vi "WinCI Open Project.vi"(8 "error in (no error)":errorcluster, 11 "configuration data":string) -> (0 "error out":errorcluster, 2 "status message":string, 3 "source control reference out":T1)   [LabVIEW 2017, in "NI_SCC_WinCI.lvlib"]
uses:
  <vilib>/SourceControl/Providers/WinCI/NI_SCC_WinCI.lvlib
  <vilib>/SourceControl/sccapi/SCCAPI Refnum.ctl
  <vilib>/SourceControl/support/SCCSup ConfigData Conv.ctl
  <vilib>/SourceControl/Providers/WinCI/WinCI SCC Project Details.ctl
  <vilib>/SourceControl/support/SCCSup Message Strings GLBL.vi
  <vilib>/SourceControl/sccapi/NI_SCC.lvlib
panel:
  out "returned project details":string
  in  "dummy refnum":T1
  out "result":i32
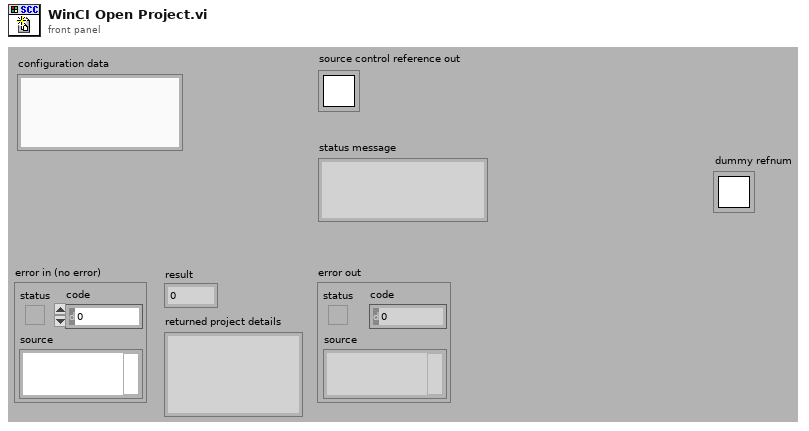
[diagram p1: front panel]
types:
  T1 = typedef "NI_SCC.lvlib/SCCAPI Refnum.ctl" = refnum<k1>
  T2 = typedef "SCCSup ConfigData Conv.ctl" = enum16{"from config data", "to config data"}
  T3 = typedef "NI_SCC_WinCI.lvlib/WinCI SCC Project Details.ctl" = cluster{"user name":string, "project name":string, "local path":string, "database name":string}
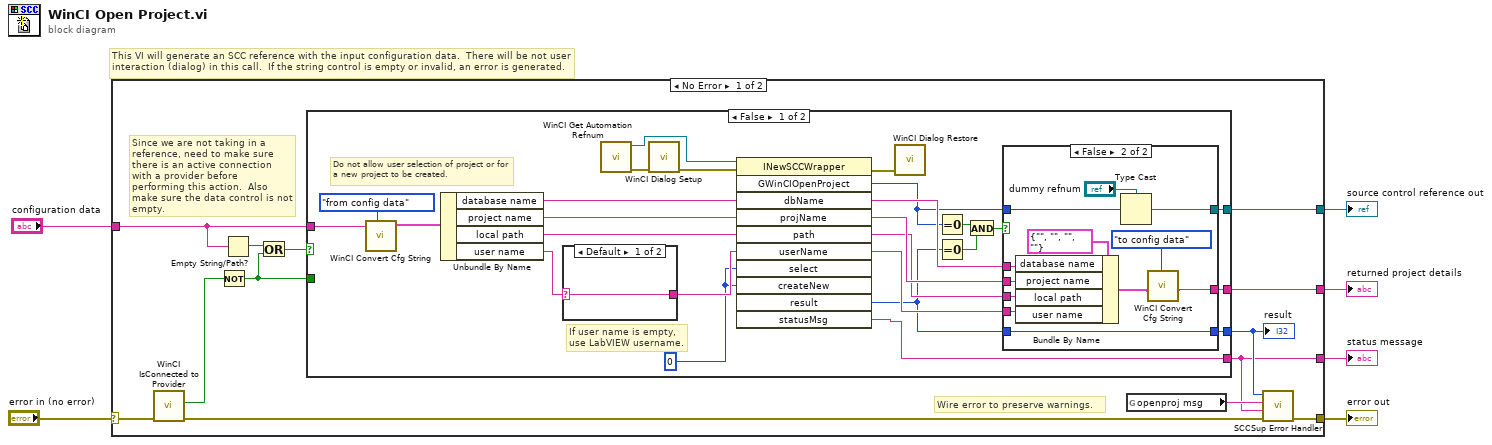
[diagram p0: block diagram]
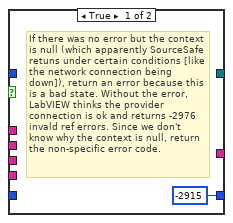
[diagram p2: hidden frame]
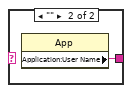
[diagram p3: hidden frame]
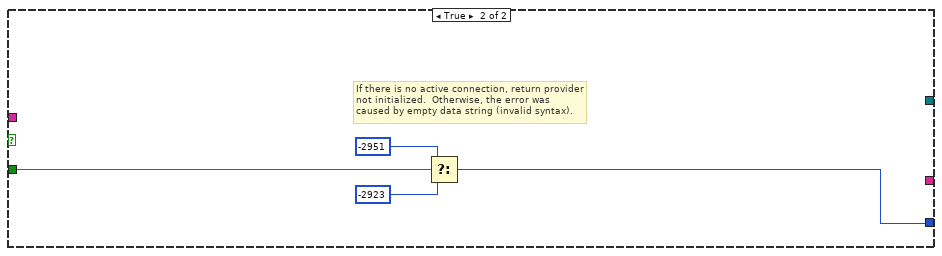
[diagram p4: hidden frame]
diagram:
  # "This VI will generate an SCC reference with the input configuration data.  There will be not user interaction (dialog) in this call.  If the string control is empty or invalid, an error is generated."
  n1 = case shown="No Error" "error in (no error)" {
    selector: "error in (no error)" -> [w8 w65]
    tunnel: [w19 _] -> w3
    tunnel: [w18 w65] -> w5
    tunnel: [w14 _] -> w4
    tunnel: "configuration data" -> [w13 _]
    tunnel: [w16 _] -> w1
    frame No Error {
      # "Since we are not taking in a reference, need to make sure there is an active connection with a provider before performing this action.  Also make sure the data control is not empty."
      # "Wire error to preserve warnings."
      n2 = call <vilib>:"WinCI IsConnected to Provider.vi"("error in (no error)"=w8) -> ("error out"=w9:errorcluster, "active connection?"=w7:bool)  [unwired: 9 out]
      n3 = Not(x=w7) -> (.not. x?=w10:bool)
      n4 = Empty String/Path?(string/path=w13) -> (empty?=w12:bool)
      n5 = Or(x=w12, y=w10) -> (x .or. y?=w11:bool)
      n6 = case shown="False" w11 {
        tunnel: [w45 _] -> w19
        tunnel: [w25 _] -> w14
        tunnel: w13 -> [w37 _]
        tunnel: [w44 _] -> w16
        tunnel: [w42 w61] -> w15
        tunnel: w10 -> [_ w64]
        frame False {
          w31 = 0
          # "If user name is empty, use LabVIEW username."
          # "Do not allow user selection of project or for a new project to be created."
          n7 = call <vilib>:"WinCI Convert Cfg String.vi"("conversion action"=SCCSup_ConfigData_Conv."from config data", "config data in"=w37) -> ("project details out"=w36:T3)  [unwired: 1 in, 8 out]
          n8 = Unbundle By Name(w36) -> ("database name"=w35:string, "project name"=w34:string, "local path"=w33:string, "user name"=w43:string)
          n9 = case shown="Default" w43 {
            selector: w43 -> [w59 _]
            tunnel: [w59 w60] -> w32
            frame Default {
            }
            frame "" {
              n10 = property class="App"() -> ("Application:User Name"=w60:string)  [unwired: 2 in, 2 out]
            }
          }
          n11 = call <vilib>:"WinCI Get Automation Refnum.vi"() -> ("error out"=w22:errorcluster, "automation refnum"=w23:refnum<k7>)  [unwired: 10 out]
          n12 = call <vilib>:"WinCI Dialog Setup.vi"("error in"=w22) -> ("error out"=w21:errorcluster)  [unwired: 10 out]
          n13 = invoke class="INewSCCWrapper" method="GWinCIOpenProject"(reference=w23, error in=w21, "dbName"=w35, "projName"=w34, "path"=w33, "userName"=w32, "select"=w31, "createNew"=w31) -> (error out=w20:errorcluster, "GWinCIOpenProject"=w24:u32, "dbName"=w30:string, "projName"=w29:string, "path"=w28:string, "userName"=w27:string, "result"=w26:i32, "statusMsg"=w25:string)  [unwired: 3 in, 3 out]
          n14 = call <vilib>:"WinCI Dialog Restore.vi"("error in"=w20) -> ()  [unwired: 11 out]
          n15 = Equal To 0?(x=w24) -> (x = 0?=w41:bool)
          n16 = Equal To 0?(x=w26) -> (x = 0?=w40:bool)
          n17 = And(x=w41, y=w40) -> (x .and. y?=w39:bool)
          n18 = case shown="False" w39 {
            tunnel: [_ w58] -> w45
            tunnel: w27 -> [_ w57]
            tunnel: w29 -> [_ w56]
            tunnel: w30 -> [_ w54]
            tunnel: w28 -> [_ w52]
            tunnel: [_ w49] -> w44
            tunnel: w26 -> [_ w51]
            tunnel: [-2915 ("result") w51] -> w42
            tunnel: w24 -> [_ w50]
            frame True {
              # "If there was no error but the context is null (which apparently SourceSafe retuns under certain conditions [like the network connection being down]), return an error because this is a bad state. Without the error, LabVIEW thinks the provider connection is ok and returns -2976 invald ref errors. Since we don't know why the context is null, return the non-specific error code."
            }
            frame False {
              n19 = Bundle By Name(cluster=T3 {"user name"="", "project name"="", "local path"="", "database name"=""} ("returned project details"), "database name"=w54, "project name"=w56, "local path"=w52, "user name"=w57) -> (w48:T3)
              n20 = Type Cast(type="dummy refnum", x=w50) -> (*(type *) &x=w58:T1)
              n21 = call <vilib>:"WinCI Convert Cfg String.vi"("conversion action"=SCCSup_ConfigData_Conv."to config data", "project details in"=w48) -> ("config data out"=w49:string)  [unwired: 1 in, 8 out]
            }
          }
        }
        frame True {
          # "If there is no active connection, return provider not initialized.  Otherwise, the error was caused by empty data string (invalid syntax)."
          n22 = Select(t=-2951 ("result"), s=w64, f=-2923 ("result")) -> (s? t:f=w61:i32)
        }
      }
      "result" <- w15
      n23 = global read "SCCSup Message Strings GLBL.vi" "openproj msg"() -> (w17:string)
      n24 = call <vilib>:"SCCSup Error Handler.vi"("error in (no error)"=w9, "additional message"=w14, "operation message"=w17, "scc error code"=w15) -> ("error out"=w18:errorcluster)  [unwired: 7 out]
    }
    frame Error {
    }
  }
  "error out" <- w5
  "status message" <- w4
  "source control reference out" <- w3
  "returned project details" <- w1
